vi "get All.vi"(8 "error in":errorcluster) -> (0 "error out":errorcluster, 3 "Data out":T1)   [LabVIEW 2015, in "App Info.lvlib"]
uses:
  App Info.lvlib
  Core Data.ctl
  Action.ctl
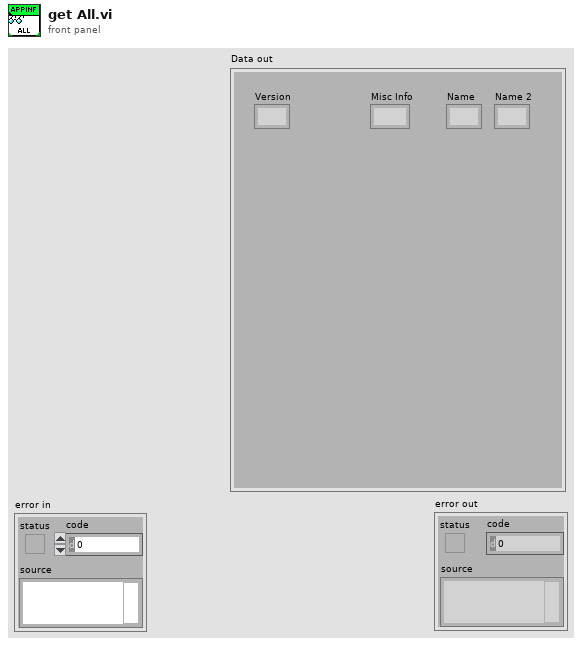
[diagram p1: front panel]
types:
  T1 = typedef "App Info.lvlib/Core Data.ctl" = cluster{"Version":string, "Misc Info":string, "Name":string, "Name 2":string}
  T2 = typedef "App Info.lvlib/Action.ctl" = enum16{"Initialise", "get All", "set Version", "set Misc Info", "set Name", "set Name 2"}
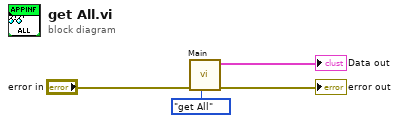
[diagram p0: block diagram]
diagram:
  n1 = call "Main.vi"("Action"=Action."get All", "error in"="error in") -> ("error out"=→"error out":errorcluster, "Data out"=→"Data out":T1)  [unwired: 8 in]
